vi "Calculate_(11)_Global_Cost_F()-1.vi"(5 "[IN] Still connect\ned tracks in group":T1, 6 "[IN] Max angle":dbl, 7 "[IN] Subtracks":T2(array[cluster]), 8 "error IN":errorcluster, 9 "[IN] Areas particles\nPrimary Detected":dbl[][](array[numeric]), 10 "[IN] Primary \n(X,Y) Detected":dbl[][](array[numeric]), 11 "[IN] Cost function":i8[](array[numeric])) -> (0 "error OUT":errorcluster, 3 "[OUT] Cost function":i8[](array[numeric]))   [LabVIEW 2013]
uses:
  <vilib>/Analysis/NI_AALBase.lvlib
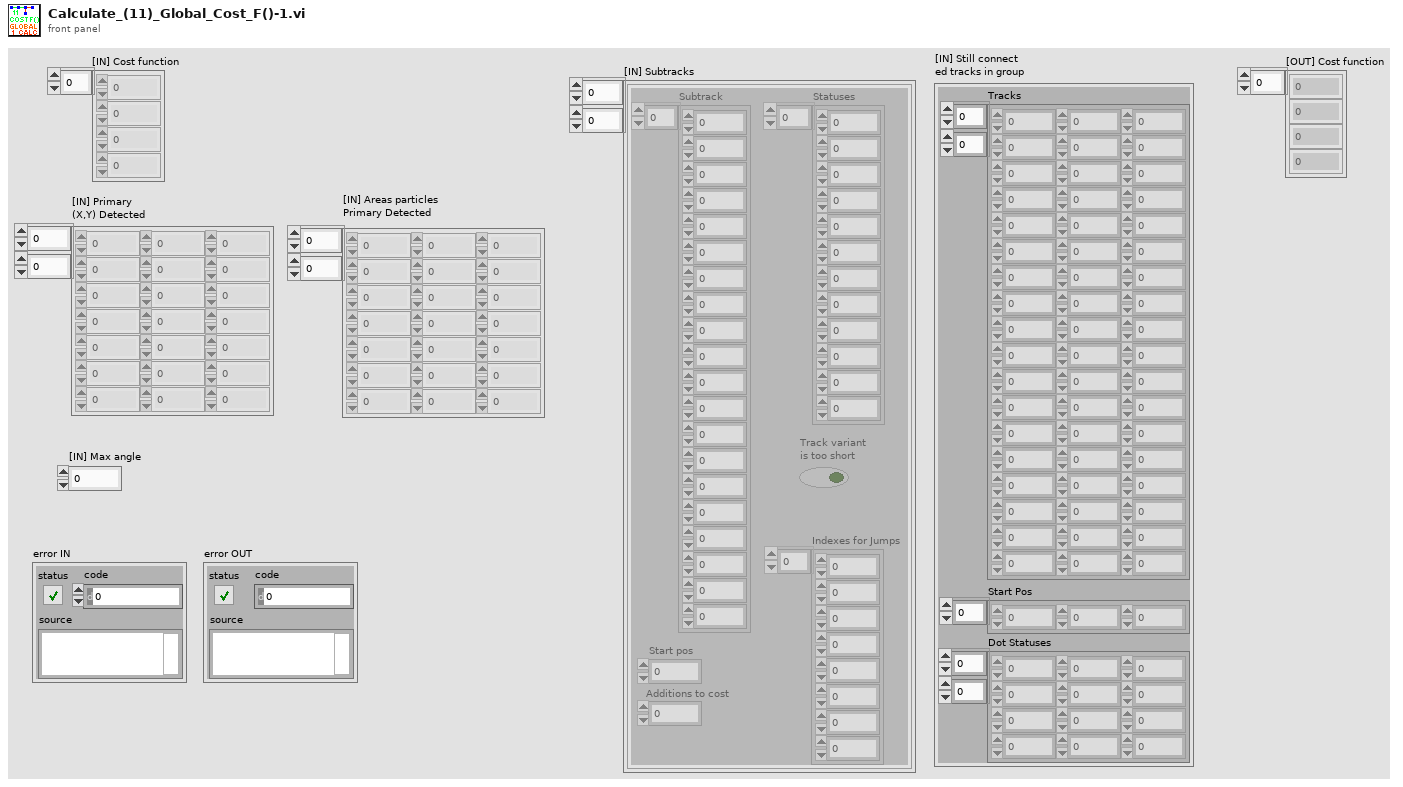
[diagram p1: front panel]
types:
  T1 = cluster{"Tracks":dbl[][], "Start Pos":i32[], "Dot Statuses":i16[][]}
  T2 = cluster{"Subtrack":dbl[], "Statuses":i16[], "Start pos":i32, "Additions to cost":i32, "Track variant \nis too short":bool, "Indexes for Jumps":i32[]}[][]
  T3 = cluster{"Subtrack":dbl[], "Statuses":i16[], "Start pos":i32, "Additions to cost":i32, "Track variant \nis too short":bool, "Indexes for Jumps":i32[]}[]
  T4 = cluster{"Subtrack":dbl[], "Statuses":i16[], "Start pos":i32, "Additions to cost":i32, "Track variant \nis too short":bool, "Indexes for Jumps":i32[]}
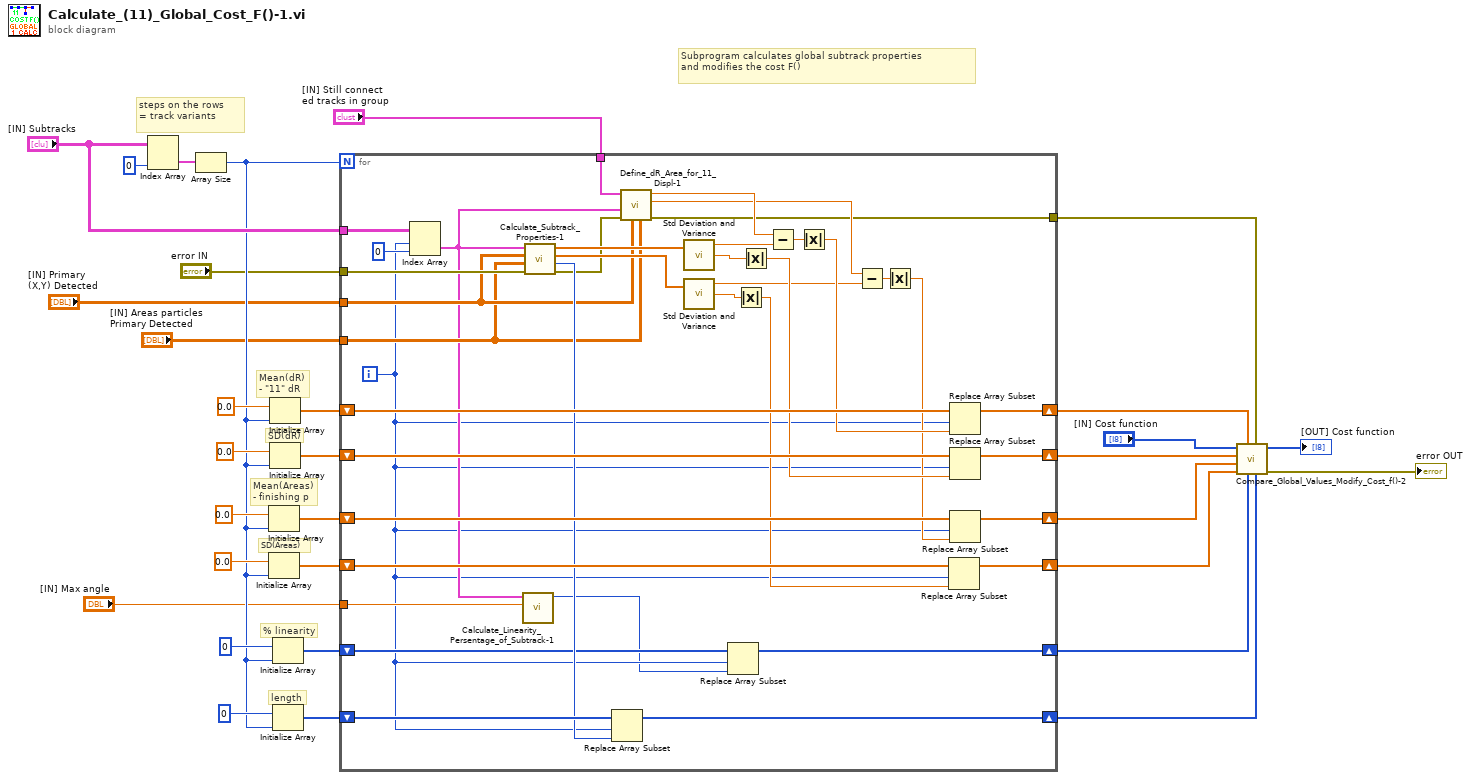
[diagram p0: block diagram]
diagram:
  # "Subprogram calculates global subtrack properties\nand modifies the cost F()"
  # "Mean(Areas)\n- finishing p"
  # "SD(Areas)"
  # "% linearity"
  # "length"
  # "Mean(dR)\n- \"11\" dR"
  # "SD(dR)"
  # "steps on the rows\n= track variants"
  n1 = Index Array(array="[IN] Subtracks", index (col)=0 ("disabled index (col)")) -> (element=w30:T3)  [unwired: 1 in]
  n2 = Array Size(array=w30) -> (size(s)=w20:i32)
  n3 = Initialize Array(0.0, w20) -> (w16:dbl[])
  n4 = Initialize Array(0.0, w20) -> (w15:dbl[])
  n5 = Initialize Array(0.0, w20) -> (w26:dbl[])
  n6 = Initialize Array(0.0, w20) -> (w25:dbl[])
  n7 = Initialize Array(u8 0, w20) -> (w11:u8[])
  n8 = Initialize Array(u8 0, w20) -> (w14:u8[])
  n9 = for {
    N: w20 -> [_]
    tunnel: "[IN] Subtracks" -> [w69]
    shift-right: [w63] -> w8
    shift-left: w26 -> [w66]
    shift-right: [w62] -> w6
    shift-left: w25 -> [w65]
    tunnel: "error IN" -> [w68]
    tunnel: "[IN] Primary \n(X,Y) Detected" -> [w48]
    tunnel: "[IN] Areas particles\nPrimary Detected" -> [w47]
    shift-right: [w56] -> w5
    shift-left: w16 -> [w61]
    shift-right: [w59] -> w4
    shift-left: w15 -> [w60]
    shift-right: [w51] -> w2
    shift-left: w14 -> [w53]
    tunnel: "[IN] Still connect\ned tracks in group" -> [w50]
    tunnel: "[IN] Max angle" -> [w38]
    shift-right: [w33] -> w3
    shift-left: w11 -> [w36]
    tunnel: [w32] -> w9
    i -> [w35]
    n10 = Index Array(array=w69, index (row)=w35, index (col)=0 ("disabled index (col)")) -> (element=w37:T4)
    n11 = call "Calculate_Linearity_Persentage_of_Subtrack-1.vi"("[IN] Max angle"=w38, "[IN] Subtrack"=w37) -> ("[OUT] Track Linearity in %"=w34:u8)  [unwired: 5 in]
    n12 = call "Calculate_Subtrack_Properties-1.vi"("error IN"=w68, "[IN] Areas particles\nPrimary Detected"=w47, "[IN] Primary \n(X,Y) Detected"=w48, "[IN] Subtrack"=w37) -> ("error OUT"=w49:errorcluster, "[OUT] Length of track"=w52:u8, "[OUT] Areas"=w64:dbl[], "[OUT] dR (displ)"=w67:dbl[])  [unwired: 2 in]
    n13 = Replace Array Subset(array=w53, new element=w52, index=w35) -> (w51:u8[])
    n14 = call "Define_dR_Area_for_11_Displ-1.vi"("[IN] Areas particles\nPrimary Detected"=w47, "[IN] Primary \n(X,Y) Detected"=w48, "error IN"=w49, "[IN] Subtrack"=w37, "[IN] Still connect\ned tracks in group"=w50) -> ("error OUT"=w32:errorcluster, "[OUT] Area of  \"11\" \ndestination point"=w41:dbl, "[OUT] dR for 11 \ndisplacement"=w45:dbl)  [unwired: 4 in]
    n15 = call <vilib>:"Std Deviation and Variance.vi"("X"=w67) -> ("mean"=w46:dbl, "standard deviation"=w58:dbl)  [unwired: 1 in, 1 out]
    n16 = call <vilib>:"Std Deviation and Variance.vi"("X"=w64) -> ("mean"=w42:dbl, "standard deviation"=w55:dbl)  [unwired: 1 in, 1 out]
    n17 = Replace Array Subset(array=w36, new element=w34, index=w35) -> (w33:u8[])
    n18 = Absolute Value(x=w55) -> (abs(x)=w54:dbl)
    n19 = Absolute Value(x=w58) -> (abs(x)=w57:dbl)
    n20 = Subtract(x=w45, y=w46) -> (x-y=w44:dbl)
    n21 = Absolute Value(x=w44) -> (abs(x)=w43:dbl)
    n22 = Subtract(x=w41, y=w42) -> (x-y=w40:dbl)
    n23 = Absolute Value(x=w40) -> (abs(x)=w39:dbl)
    n24 = Replace Array Subset(array=w60, new element=w54, index=w35) -> (w59:dbl[])
    n25 = Replace Array Subset(array=w66, new element=w43, index=w35) -> (w63:dbl[])
    n26 = Replace Array Subset(array=w65, new element=w57, index=w35) -> (w62:dbl[])
    n27 = Replace Array Subset(array=w61, new element=w39, index=w35) -> (w56:dbl[])
  }
  n28 = call "Compare_Global_Values_Modify_Cost_f()-2.vi"("[IN] Lengths"=w2, "error IN"=w9, "[IN] Linearity"=w3, "[IN] Array of Mean\n(dR) - Problem dR"=w8, "[IN] SD(Areas)"=w4, "[IN] Array of Mean(Areas)\n - Problem finish Area"=w5, "[IN] SD(dR)"=w6, "[IN] Cost function"="[IN] Cost function") -> ("error OUT"=→"error OUT":errorcluster, "[OUT] Cost function"=→"[OUT] Cost function":i8[])  [unwired: 2 in]
